vi "Check_For_Gate_Resistor.vi"(8 "error in":errorcluster, 10 "Device Type":string, 11 "FET Test Configuration":string) -> (0 "error out":errorcluster, 1 "Frequency":string, 3 "Test Comment":string)   [LabVIEW 2020]
uses:
  Global 1.vi
panel:
  out "CapDeltaPercent":dbl[](array[numeric]) format="%_6g"
  out "CapValue":dbl[](array[numeric]) format="%_6g"
  out "Capacitance Data (in pF)":dbl format="%_6g"
  in  "Keystate":string
  # "A2B2C1F17H0I1M2R31S0T1E"
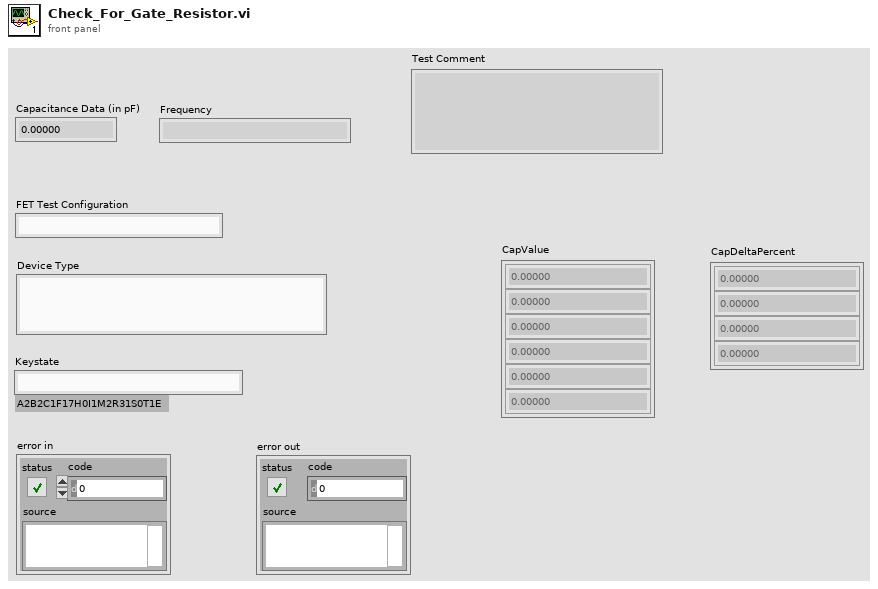
[diagram p1: front panel]
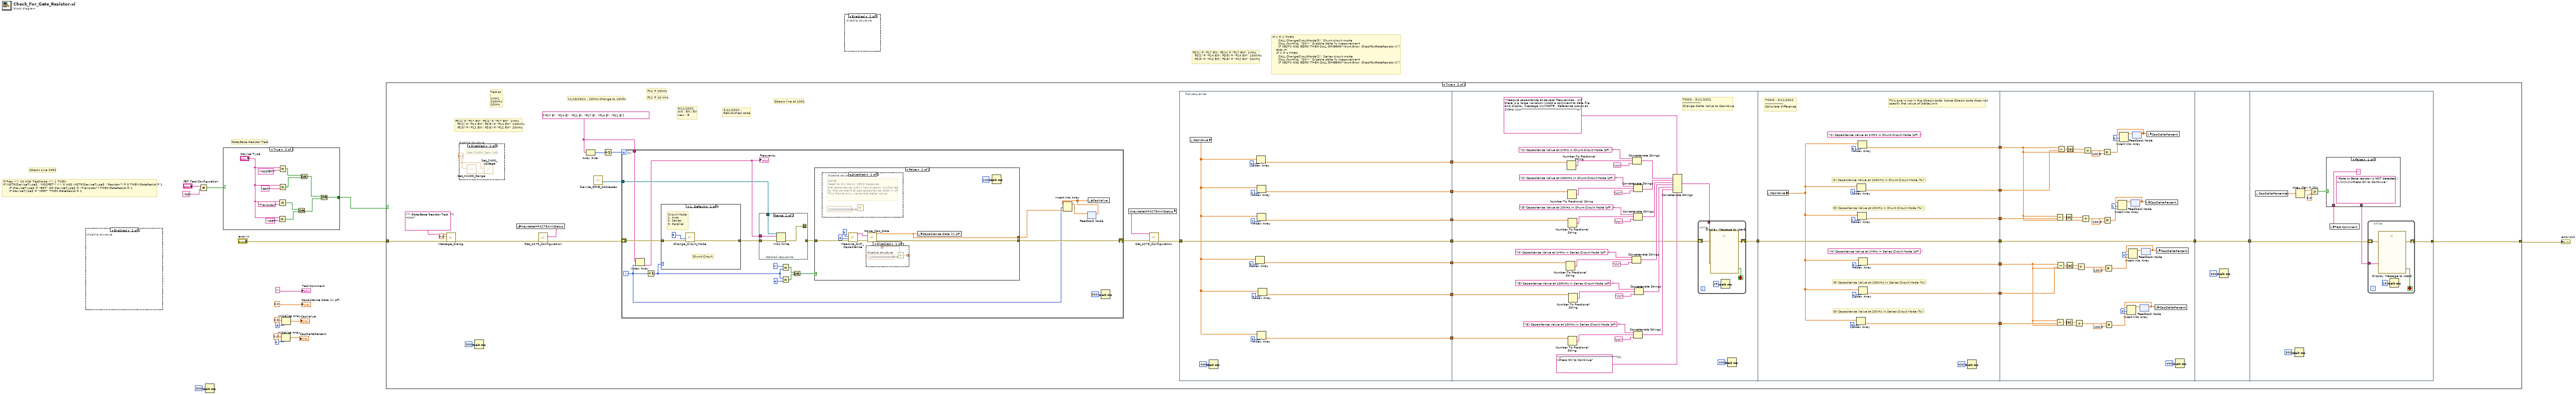
[diagram p0: block diagram]
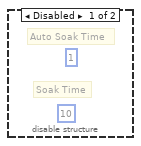
[diagram p2: hidden frame]
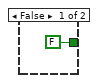
[diagram p3: hidden frame]
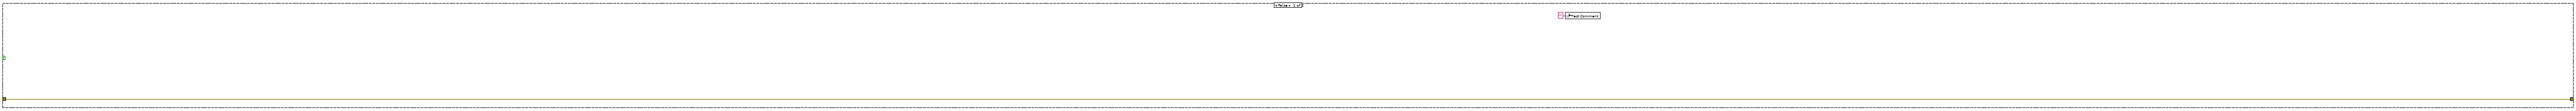
[diagram p4: hidden frame]
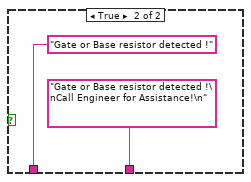
[diagram p6: hidden frame]
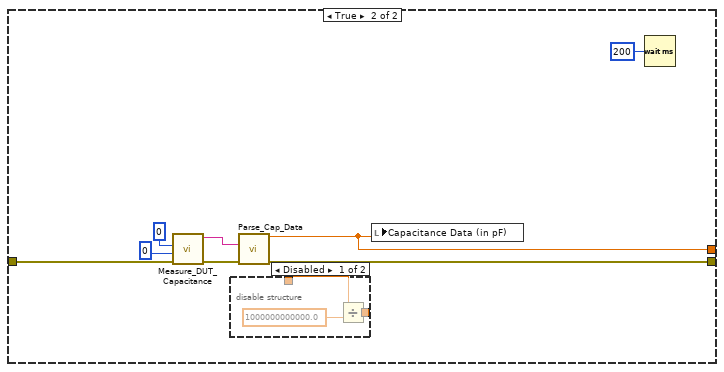
[diagram p9: hidden frame]
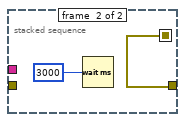
[diagram p11: hidden frame]
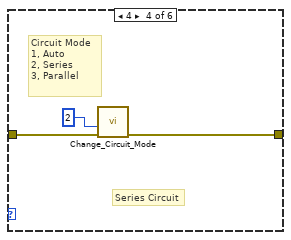
[diagram p14: hidden frame]
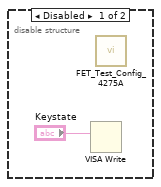
[diagram p17: hidden frame]
diagram:
  # "IF X = 1 THEN\n      CALL ChangeCircuitMode(3) ' Shunt circuit mode\n      CALL Ibwrt(lcz, \"D0\") ' Disable delta % measurement\n      IF (IBSTA AND EERR) THEN CALL GPIBERR(\"Ibwrt Error, CheckForGateResistor 1\")\n    END IF\n    IF X = 4 THEN\n      CALL ChangeCircuitMode(2) ' Series circuit mode\n      CALL Ibwrt(lcz, \"D0\") ' Disable delta % measurement\n      IF (IBSTA AND EERR) THEN CALL GPIBERR(\"Ibwrt Error, CheckForGateResistor 2\")"
  # "F$(1) = \"F17 EN\": F$(4) = \"F17 EN\"' 1MHz\n  F$(2) = \"F14 EN\": F$(5) = \"F14 EN\"' 100KHz\n  F$(3) = \"F12 EN\": F$(6) = \"F12 EN\"' 20KHz"
  # "Qbasic Line 2051"
  # "IF Freq <> 10 AND TestMode <> 1 THEN\nIF INSTR(DeviceType$, \"MOSFET\") <> 0 AND INSTR(DeviceType$, \"Resistor\") = 0 THEN GateResist = 1\n      IF (DeviceType$ = \"BRT\" OR DeviceType$ = \"Transistor\") THEN GateResist = 1\n      IF DeviceType$ = \"IGBT\" THEN GateResist = 1"
  # "Gate/Base Resistor Test"
  n1 = disable-structure shown="Enabled" {
    frame Disabled {
      n2 = VISA Write(write buffer="Keystate") -> ()  [unwired: 2 in, 3 out]
      n3 = call "FET_Test_Config_4275A.vi"() -> ()  [unwired: 11 in, 1 out]
    }
    frame Enabled {
    }
  }
  n4 = Not Equal?(x="FET Test Configuration", y="RG") -> (x != y?=w9:bool)
  n5 = Wait (ms)(milliseconds to wait=u32 300) -> ()  [unwired: 1 out]
  n6 = case shown="True" w9 {
    tunnel: [FALSE w18] -> w13
    frame False {
    }
    frame True {
      n7 = Equal?(x="Device Type", y="IGBT") -> (x = y?=w21:bool)
      n8 = Equal?(x="Device Type", y="Transistor") -> (x = y?=w22:bool)
      n9 = Equal?(x="Device Type", y="MOSFET") -> (x = y?=w24:bool)
      n10 = Equal?(x="Device Type", y="BRT") -> (x = y?=w23:bool)
      n11 = Or(x=w22, y=w21) -> (x .or. y?=w19:bool)
      n12 = Or(x=w24, y=w23) -> (x .or. y?=w20:bool)
      n13 = Or(x=w20, y=w19) -> (x .or. y?=w18:bool)
    }
  }
  n14 = Initialize Array(0.0 ("element"), 4 ("dimension size")) -> (→"CapDeltaPercent":dbl[])
  n15 = Initialize Array(0.0 ("element"), 6 ("dimension size")) -> (→"CapValue":dbl[])
  n16 = case shown="True" w13 {
    tunnel: "error in" -> [w31 w35]
    tunnel: [w31 w62] -> w14
    frame False {
      n17 = local write "Test Comment"("" ("Test Comment")) -> ()
    }
    frame True {
      w47 = string[] ["F17 E", "F14 E", "F11 E", "F17 E", "F14 E", "F11 E"]
      # "3/11/2022:\nRefurbished code"
      # "3/11/2022\nold : EN / EX\nnew : E"
      # "F$(1) = \"F17 EN\": F$(4) = \"F17 EN\"' 1MHz\n  F$(2) = \"F14 EN\": F$(5) = \"F14 EN\"' 100KHz\n  F$(3) = \"F12 EN\": F$(6) = \"F12 EN\"' 20KHz"
      # "Test at :\n1MHZ\n100kHz\n10kHz"
      # "F12 = 20kHz"
      # "F11 = 10 KHz"
      # "11/18/2021 : 20kHz Change to 10kHz"
      # "Qbasic line at 1001"
      n18 = call "Message_dialog.vi"("error in (no error)"=w35, "set delay"=3.0, "String"="** Gate/Base Resistor Test  **\n\n\n") -> ("error out"=w34:errorcluster)  [unwired: 8 in]
      n19 = disable-structure shown="Disabled" {
        frame Disabled {
          w65 = 0.0
          # "Set K2400 Zero Volt"
          n20 = call "Set_K2400_Range.vi"("Desired Voltage"=w65) -> ("error out"=w66:errorcluster)  [unwired: 10 in]
          n21 = call "Set_2400_Voltage.vi"("error in"=w66, "Voltage"=w65) -> ("error out"=w64:errorcluster)  [unwired: 8 in]
        }
        frame Enabled {
        }
      }
      n22 = Wait (ms)(milliseconds to wait=u32 300) -> ()  [unwired: 1 out]
      n23 = call "Get_4275_Configuration.vi"("error in"=w34) -> ("error out"=w58:errorcluster, "Keystate"=w59:string)  [unwired: 9 in]
      n24 = global write "Global 1.vi" "KeystateHP4275AInitSetup"(w59) -> ()
      n25 = Array Size(array=w47) -> (size(s)=w46:i32)
      n26 = call "Device_GPIB_Addresses.vi"() -> ("HP 4275A Address"=w63:refnum<visa-resource-name>)  [unwired: 9 in, 2 out]
      n27 = Increment(x=w46) -> (x+1=w45:i32)
      n28 = for {
        N: w45 -> [_]
        tunnel: w63 -> [w208]
        shift-right: [w202] -> w60
        shift-left: w58 -> [w205]
        tunnel: w47 -> [w199]
        i -> [w200]
        n29 = Index Array(array=w199, index=w200) -> (element=w198:string)
        "Frequency" <- w198
        n30 = Increment(x=w200) -> (x+1=w204:i32)
        n31 = case shown="1, Default" w204 {
          tunnel: w205 -> [w247 w248 w249 w252 w253 w254]
          tunnel: [w245 w248 w249 w250 w253 w254] -> w215
          frame 1, Default {
            # "Shunt Circuit"
            # "Circuit Mode\n1, Auto\n2, Series\n3, Parallel"
            n32 = call "Change_Circuit_Mode.vi"("Error In"=w247, "Circuit Mode\n1, Auto\n2, Series\n3, Parallel"=3 ("Circuit Mode\n1, Auto\n2, Series\n3, Parallel")) -> ("error out"=w245:errorcluster)  [unwired: 9 in]
          }
          frame 2 {
          }
          frame 3 {
          }
          frame 4 {
            # "Series Circuit"
            # "Circuit Mode\n1, Auto\n2, Series\n3, Parallel"
            n33 = call "Change_Circuit_Mode.vi"("Error In"=w252, "Circuit Mode\n1, Auto\n2, Series\n3, Parallel"=2 ("Circuit Mode\n1, Auto\n2, Series\n3, Parallel")) -> ("error out"=w250:errorcluster)  [unwired: 9 in]
          }
          frame 5 {
          }
          frame 6 {
          }
        }
        n34 = stacked-sequence {
          seq-local: [w239 _] -> [_ w243]
          tunnel: w198 -> [w241 _]
          tunnel: w215 -> [w240 _]
          tunnel: [_ w243] -> w209
          tunnel: w208 -> [w242 _]
          frame #0 {
            n35 = VISA Write(VISA resource name=w242, write buffer=w241, error in (no error)=w240) -> (error out=w239:errorcluster)  [unwired: 2 out]
          }
          frame #1 {
            n36 = Wait (ms)(milliseconds to wait=u32 3000) -> ()  [unwired: 1 out]
          }
        }
        n37 = Equal?(x=1, y=w204) -> (x = y?=w213:bool)
        n38 = Equal?(x=w204, y=4) -> (x = y?=w214:bool)
        n39 = Or(x=w213, y=w214) -> (x .or. y?=w210:bool)
        n40 = case shown="False" w210 {
          tunnel: w209 -> [w219 w233]
          tunnel: [w218 w232] -> w202
          tunnel: [w216 w228] -> w201
          frame False {
            n41 = disable-structure shown="Disabled" {
              frame Disabled {
                # "NOTE : \nNeed to divide by 1E12 because\nthe capacitance subVI has already multiplied\nby the constant to get capacitance data in pF\nThis frame only wants the delta value"
                n42 = Divide(y=1000000000000.0) -> ()  [unwired: 1 in, 1 out]
              }
              frame Enabled {
              }
            }
            n43 = call "Measure_DUT_Capacitance.vi"("error in"=w219, "SoakTime"=u16 0, "AutoSoakFlag"=u16 0) -> ("error out"=w222:errorcluster, "Measure$"=w217:string)  [unwired: 5 in, 2 out]
            n44 = disable-structure shown="Disabled" {
              disable-tunnel: _ -> [w226 _]
              disable-tunnel: [w224 _] -> _
              frame Disabled {
                n45 = Divide(x=w226, y=1000000000000.0) -> (x/y=w224:dbl)
              }
              frame Enabled {
              }
            }
            n46 = call "Parse_Cap_Data.vi"("Measure$"=w217, "error in"=w222) -> ("Capacitance Data (in pF)"=w216:dbl, "error out"=w218:errorcluster)  [unwired: 8 in, 4 out]
            n47 = local write "Capacitance Data (in pF)"(w216) -> ()
            n48 = Wait (ms)(milliseconds to wait=u32 200) -> ()  [unwired: 1 out]
          }
          frame True {
            n49 = call "Measure_DUT_Capacitance.vi"("error in"=w233, "SoakTime"=u16 0, "AutoSoakFlag"=u16 0) -> ("error out"=w235:errorcluster, "Measure$"=w229:string)  [unwired: 5 in, 2 out]
            n50 = disable-structure shown="Disabled" {
              disable-tunnel: _ -> [w238 _]
              disable-tunnel: [w237 _] -> _
              frame Disabled {
                n51 = Divide(x=w238, y=1000000000000.0) -> (x/y=w237:dbl)
              }
              frame Enabled {
              }
            }
            n52 = call "Parse_Cap_Data.vi"("Measure$"=w229, "error in"=w235) -> ("Capacitance Data (in pF)"=w228:dbl, "error out"=w232:errorcluster)  [unwired: 8 in, 4 out]
            n53 = local write "Capacitance Data (in pF)"(w228) -> ()
            n54 = Wait (ms)(milliseconds to wait=u32 200) -> ()  [unwired: 1 out]
          }
        }
        n55 = feedback #1() -> (w206:dbl[])  [unwired: 1 in]
        n56 = Insert Into Array(array=w206, index=w200, new element=w201) -> (w207:dbl[])
        n57 = feedback-in #1(w207) -> ()
        n58 = local write "CapValue"(w206) -> ()
        n59 = Wait (ms)(milliseconds to wait=u32 300) -> ()  [unwired: 1 out]
      }
      n60 = global read "Global 1.vi" "KeystateHP4275AInitSetup"() -> (w61:string)
      n61 = call "Set_4275_Configuration.vi"("error in"=w60, "Keystate"=w61) -> ("error out"=w37:errorcluster)  [unwired: 9 in]
      n62 = flat-sequence {
        tunnel: [w73] -> w43
        tunnel: [w72] -> w42
        tunnel: [w71] -> w41
        tunnel: [w70] -> w40
        tunnel: [w69] -> w39
        tunnel: [w68] -> w38
        tunnel: w37 -> [w67]
        tunnel: [w67] -> w36
        tunnel: [w84] -> w44
        tunnel: w43 -> [w100]
        tunnel: w42 -> [w97]
        tunnel: w41 -> [w94]
        tunnel: w40 -> [w91]
        tunnel: w39 -> [w88]
        tunnel: w38 -> [w85]
        tunnel: w36 -> [w83]
        tunnel: w44 -> [w131]
        tunnel: [w131] -> w56
        tunnel: [w129] -> w55
        tunnel: [w128] -> w54
        tunnel: [w127] -> w53
        tunnel: [w125] -> w52
        tunnel: [w124] -> w51
        tunnel: [w123] -> w50
        tunnel: w56 -> [w177]
        tunnel: [w177] -> w49
        tunnel: w55 -> [w171]
        tunnel: w54 -> [w153]
        tunnel: w53 -> [w169]
        tunnel: w52 -> [w150]
        tunnel: w51 -> [w157]
        tunnel: w50 -> [w156]
        tunnel: w49 -> [w179]
        tunnel: [w179] -> w48
        tunnel: [w185] -> w62
        tunnel: w48 -> [w186]
        frame #0 {
          n63 = local read "CapValue"() -> (w75:dbl[])
          n64 = Wait (ms)(milliseconds to wait=u32 400) -> ()  [unwired: 1 out]
          n65 = Index Array(array=w75, index=3) -> (element=w71:dbl)
          n66 = Index Array(array=w75, index=0) -> (element=w68:dbl)
          n67 = Index Array(array=w75, index=1) -> (element=w69:dbl)
          n68 = Index Array(array=w75, index=2) -> (element=w70:dbl)
          n69 = Index Array(array=w75, index=5) -> (element=w73:dbl)
          n70 = Index Array(array=w75, index=4) -> (element=w72:dbl)
        }
        frame #1 {
          # "TODO : 3/11/2022\n------------------\nChange Delta Value to CapValue"
          n71 = Number To Fractional String(number=w94) -> (F-format string=w107:string)  [unwired: 3 in]
          n72 = Number To Fractional String(number=w85) -> (F-format string=w110:string)  [unwired: 3 in]
          n73 = Number To Fractional String(number=w88) -> (F-format string=w105:string)  [unwired: 3 in]
          n74 = Number To Fractional String(number=w91) -> (F-format string=w106:string)  [unwired: 3 in]
          n75 = Number To Fractional String(number=w100) -> (F-format string=w109:string)  [unwired: 3 in]
          n76 = Number To Fractional String(number=w97) -> (F-format string=w108:string)  [unwired: 3 in]
          n77 = Concatenate Strings("(4) Capacitance Value at 1MHz in Series Circuit Mode (pF) : ", w107, "\r\n") -> (w114:string)
          n78 = Concatenate Strings("(1) Capacitance Value at 1MHz in Shunt Circuit Mode (pF) : ", w110, "\r\n") -> (w113:string)
          n79 = Concatenate Strings("(2) Capacitance Value at 100KHz in Shunt Circuit Mode (pF) : ", w105, "\r\n") -> (w111:string)
          n80 = Concatenate Strings("(3) Capacitance Value at 10KHz in Shunt Circuit Mode (pF) : ", w106, "\r\n") -> (w112:string)
          n81 = Concatenate Strings("(6) Capacitance Value at 10KHz in Series Circuit Mode (pF) : ", w109, "\r\n") -> (w116:string)
          n82 = Concatenate Strings("(5) Capacitance Value at 100KHz in Series Circuit Mode (pF) : ", w108, "\r\n") -> (w115:string)
          n83 = Concatenate Strings("Measure capacitance at several frequencies.  \nIf there is a large variation,\nAdd a comment to data file and display message.\n\n(NOTE : Reference occurs at 1MHz) \n\n*************************************\n" ("Message"), w113, w111, w112, w114, w115, w116, "\n*************************************\n\nPress OK to Continue" ("string")) -> (w117:string)
          n84 = while {
            tunnel: w117 -> [w121]
            shift-right: [w120] -> w84
            shift-left: w83 -> [w122]
            stop <- w119 stop-if-true
            n85 = call "Display Message to User3"("error in (no error)"=w122, "Message"=w121) -> ("error out"=w120:errorcluster, "OK"=w119:bool)  [unwired: 8 in]
            n86 = Wait (ms)(milliseconds to wait=u32 25) -> ()  [unwired: 1 out]
          }
          n87 = Wait (ms)(milliseconds to wait=u32 400) -> ()  [unwired: 1 out]
        }
        frame #2 {
          (unwired) "(4) Capacitance Value at 1MHz in Series Circuit Mode (pF) : "
          (unwired) "(1) Capacitance Value at 1MHz in Shunt Circuit Mode (pF) : "
          # "TODO : 3/11/2022\n------------------\nCalculate difference"
          # "This one is not in the Qbasic code, bcoze Qbasic code does not\nspecify the value of DeltaLimit"
          # "(6) Capacitance Value at 20KHz in Series Circuit Mode (%) :"
          # "(5) Capacitance Value at 100KHz in Series Circuit Mode (%) :"
          # "(3) Capacitance Value at 20KHz in Shunt Circuit Mode (%) :"
          # "(2) Capacitance Value at 100KHz in Shunt Circuit Mode (%) :"
          n88 = local read "CapValue"() -> (w126:dbl[])
          n89 = Index Array(array=w126, index=5) -> (element=w123:dbl)
          n90 = Index Array(array=w126, index=1) -> (element=w127:dbl)
          n91 = Index Array(array=w126, index=2) -> (element=w129:dbl)
          n92 = Index Array(array=w126, index=0) -> (element=w128:dbl)
          n93 = Index Array(array=w126, index=3) -> (element=w125:dbl)
          n94 = Index Array(array=w126, index=4) -> (element=w124:dbl)
          n95 = Wait (ms)(milliseconds to wait=u32 400) -> ()  [unwired: 1 out]
        }
        frame #3 {
          n96 = Subtract(x=w153, y=w171) -> (x-y=w176:dbl)
          n97 = Subtract(x=w150, y=w156) -> (x-y=w158:dbl)
          n98 = Subtract(x=w150, y=w157) -> (x-y=w161:dbl)
          n99 = Subtract(x=w153, y=w169) -> (x-y=w173:dbl)
          n100 = Absolute Value(x=w176) -> (abs(x)=w154:dbl)
          n101 = Absolute Value(x=w158) -> (abs(x)=w151:dbl)
          n102 = Absolute Value(x=w161) -> (abs(x)=w152:dbl)
          n103 = Absolute Value(x=w173) -> (abs(x)=w155:dbl)
          n104 = Divide(x=w151, y=w150) -> (x/y=w139:dbl)
          n105 = Divide(x=w152, y=w150) -> (x/y=w141:dbl)
          n106 = Divide(x=w154, y=w153) -> (x/y=w143:dbl)
          n107 = Divide(x=w155, y=w153) -> (x/y=w145:dbl)
          n108 = Multiply(x=w145, y=100.0) -> (x*y=w144:dbl)
          n109 = Multiply(x=w143, y=100.0) -> (x*y=w142:dbl)
          n110 = Multiply(x=w141, y=100.0) -> (x*y=w140:dbl)
          n111 = Multiply(x=w139, y=100.0) -> (x*y=w138:dbl)
          n112 = feedback #2() -> (w175:dbl[])  [unwired: 1 in]
          n113 = Insert Into Array(array=w175, index=1, new element=w142) -> (w168:dbl[])
          n114 = feedback-in #2(w168) -> ()
          n115 = feedback #3() -> (w174:dbl[])  [unwired: 1 in]
          n116 = Insert Into Array(array=w174, index=0, new element=w144) -> (w167:dbl[])
          n117 = feedback-in #3(w167) -> ()
          n118 = feedback #4() -> (w159:dbl[])  [unwired: 1 in]
          n119 = Insert Into Array(array=w159, index=3, new element=w138) -> (w164:dbl[])
          n120 = feedback-in #4(w164) -> ()
          n121 = feedback #5() -> (w160:dbl[])  [unwired: 1 in]
          n122 = Insert Into Array(array=w160, index=2, new element=w140) -> (w165:dbl[])
          n123 = feedback-in #5(w165) -> ()
          n124 = local write "CapDeltaPercent"(w175) -> ()
          n125 = local write "CapDeltaPercent"(w174) -> ()
          n126 = local write "CapDeltaPercent"(w159) -> ()
          n127 = local write "CapDeltaPercent"(w160) -> ()
          n128 = Wait (ms)(milliseconds to wait=u32 400) -> ()  [unwired: 1 out]
        }
        frame #4 {
          n129 = Wait (ms)(milliseconds to wait=u32 300) -> ()  [unwired: 1 out]
        }
        frame #5 {
          n130 = local read "CapDeltaPercent"() -> (w183:dbl[])
          n131 = Wait (ms)(milliseconds to wait=u32 300) -> ()  [unwired: 1 out]
          n132 = Array Max & Min(array=w183) -> (max value=w182:dbl)  [unwired: 3 out]
          n133 = Greater?(x=w182, y=5.0) -> (0:w180:bool)
          n134 = case shown="False" w180 {
            tunnel: ["Gate or Base resistor is NOT detected \n:)\n\n\n\nPress OK to Continue." "Gate or Base resistor detected !\nCall Engineer for Assistance!\n"] -> w187
            tunnel: ["" "Gate or Base resistor detected !"] -> w188
            frame False {
            }
            frame True {
            }
          }
          n135 = local write "Test Comment"(w188) -> ()
          n136 = while {
            tunnel: w187 -> [w193]
            shift-right: [w191] -> w185
            shift-left: w186 -> [w192]
            stop <- w190 stop-if-true
            n137 = call "Display Message to User2"("error in (no error)"=w192, "Message"=w193) -> ("error out"=w191:errorcluster, "OK"=w190:bool)  [unwired: 8 in]
            n138 = Wait (ms)(milliseconds to wait=u32 25) -> ()  [unwired: 1 out]
          }
        }
      }
    }
  }
  "error out" <- w14
  n139 = disable-structure shown="Enabled" {
    frame Disabled {
      (unwired) u16 10 ("SoakTime")
      (unwired) u16 1 ("AutoSoakFlag")
      # "Auto Soak Time"
      # "Soak Time"
    }
    frame Enabled {
    }
  }
  "Test Comment" <- "" ("Test Comment")
  "Capacitance Data (in pF)" <- 0.0 ("Capacitance Data (in pF)")
